vi "AppInit.vi"(10 "path":path, 11 "Changelog":string caption="App Ver") -> (0 "error out":errorcluster)   [LabVIEW 2016]
doc: "Init Host application"
uses:
  tools/Windows/Windows.ExitAction.ctl
  tools/EventLog/EventLog.Buffer.Action.ctl
  tools/Translator/Translator.Message.ctl
  Global/ApplicationGlobal.vi
  Station/Station.Global.vi
  tools/EventLog/EventLog.New(single).vi
  tools/Config/Config.Global.vi
panel:
  out "idx":i32
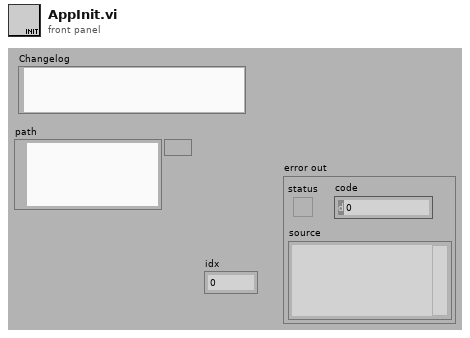
[diagram p1: front panel]
types:
  T1 = enum32{"Invalid", "Standard", "Closed", "Hidden", "Minimized", "Maximized"}
  T2 = typedef "Windows.ExitAction.ctl" = enum16{"Log off from PC", "Shut Down PC", "Reboot PC", "Close Program"}
  T3 = typedef "EventLog.Buffer.Action.ctl" = enum16{"init", "re-init", "clear", "set translator", "add", "get", "get unsaved"}
  T4 = typedef "Translator.Message.ctl" = enum16{"-", "Event confirmed", "Log out", "Log in", "Shutdown", "Cancel", "Start", "Begin time", "End time", "Duration", "Service Mode", "Ignore Results", "Serial Format", "On", "Off", "OK", "NOK", "NOK %s", "Home", "Work", "Close", "Open", "In progress...", "Missing", "Empty", "Hardware failure", "Initial", "Default", "Total", "Out of range", "Free disk space is below 1GB - contact technician", "Error %d >> %s", "Error %d >> %s >> %s", "Msg %d >> %s", "Laser msg %d %s", "Laser cmd error %s %d", "Laser cmd failed %s", "Laser cmd warning %s", "Laser disconnected", "Laser status %s", "Laser already started", "Laser job unkonwn %s", "Laser job missing %s", "Laser job select failure %s", "Unable to start laser printing (%s)", "Unable to stop laser printing (%s)", "Laser marking aborted", "Laser marking timeout", "Unable to reset Laser Interlock (%s)", "Unable to trigger Laser. Laser not ready (%s)", "Laser job '%s' coordinates not configured", "Starting %s", "Quitting %s", "Configured", "Initializing", "Quitting", "Loading", "Loaded %d results", "Loaded %d events", "Running", "Stopped", "Summary", "Laser", "Do you want to continue?", "Do you want to delete the configuration?", "The configuration is being used by an order. Unable to delete!", "Press confirm button", "Station is not based. Do you want to exit?", "Station requires changeover. Do you want to run the test?", "Test options are not set as default. Do you want to continue?", "Formatting of WabcoNo is disabled. Do you want to continue?", "Product not detected. Do you want to continue?", "Product scan failed. Do you want to continue?", "Calibration", "Log out?", "System", "All", "IDLE", "Translating...%s", "Not found", "Alarm %s", "Run", "Skip", "Abort", "Repeat", "Please wait...", "Database disconnected", "Database disconnected - changeover disabled!", "Login to database successful", "Login to database failed: %d; %s", "Unable to check the product status of reference %d - database disconnected", "Unable to set the product status of reference %d - database disconnected", "Variant file backup %s", "Read variant (%s)", "Result", "Station armed!", "Station requires changeover!", "Select reference number...", "EMERGENCY BUTTON - press Control button", "EMERGENCY DOOR - press Control button", "Resetting Emergency...", "Unable to reset safety circuit - Emergency Button pressed", "Unable to reset safety circuit - Emergency Side Door open", "Station not based", "Station based", "Station not empty", "Station basing...", "No order", "Press Start to begin new order", "Scanning new order", "Order NOK. Correct or scan again", "Order OK. Press Accept", "Order ready", "Revolver incorrect", "Fork incorrect", "Revolver missing", "Revolver empty", "Container missing", "Offline results", "Offline statistics", "Updating statistics %.1f %%", "DMC Configurator", "Door open", "Close the front door", "Press start button", "Done. Open the front door", "Running...", "Running...%.1f %%", "Pause %s", "Pause %s. NOK container missing", "Pause %s. OK container missing", "Pause %s. Revolver empty", "Pause %s. Revolver missing", "Pause %s. Revolver incorrect", "Pause %s. Fork missing", "Pause %s. Fork incorrect", "Pause %s. Too many failures", "Pause %s. Unloading failure", "Pause %s. One slot is not working", "Pause %s. Part order is done. Empty OK container", "Pause %s. Unable to move product to slot", "Pause %s. Unable to move back product pusher", "Pause %s. Unable to lift product", "Pause %s. Unable to move back product lifter", "Pause %s. Unable to move product arm to Work", "Pause %s. Unable to move product arm to NOK", "Pause %s. Unable to move product arm to OK", "Pause %s. Unable to unsuck the NOK product", "Pause %s. Unable to drop the NOK product", "Pause %s. Product OK missing", "Pause %s. Unable to unsuck the OK product", "Pause %s. Unable to drop the OK product", "Stopping...", "File '%s' is missing", "File '%s' is broken", "File '%s' is running", "Log file started (%s)", "Log file ended (%s)", "Log file stopped (%s)", "Log file ignored (%s)", "Log file exported (%s)", "Log file export failed (%s)", "Wrong serial number in log file", "Wrong reference number in log file", "Test steps are missing", "%s = %.3f", "Process param '%s' not found in DB", "Process param '%s' wrong order", "Process param '%s' value %.3f out of limits (%.3f; %.3f)", "Step%d param '%s' not found in DB", "Step%d param '%s' wrong order", "Step%d param '%s' value %.3f out of limits (%.3f; %.3f)", "Step%d EV '%s' not found in DB", "Step%d EV '%s' wrong order", "\"%s\" not found in DB", "\"%s\" wrong order", "\"%s\" value %.3f out of limits (%.3f; %.3f)", "\"%s\" not found in software", "Process init (%s)", "Process started", "Process restarted", "Process run", "Process done", "Process done - remove OK container", "Process aborted", "Process aborted at work", "Process aborted at home", "Process error", "Process error at home", "Process error at work", "Process close", "Process pause", "Process continue", "Process door open", "Process door close", "Process pause at slot %s due to %s", "Select plate from the order to process", "Do you want to start the process?", "Do you want to continue the process?", "There is unfinished order. Do you want to put the new order?", "Product %s %d OK", "Product %s %d NOK", "Unable to unload the slot %s. Product missing in the slot", "Unable to unload the slot %s. Product already in the arm", "Unable to accept the product as OK. Product missing in slot %s", "Unable to accept the product as OK. Product could not drop into the container at slot %s", "Unable to accept the product as NOK. Product could not drop into the container at slot %s", "Scan failed. Error %s", "Scan failed. Scanner disconnected", "Scan failed. Wrong Wabco number %d, limit (%d,%d)", "Scan failed. Wrong serial number %d, limit (%d,%d)", "Scan failed. Wrong date %d, limit (%d,%d)", "Scan failed. Wrong product wabco number %d (expected %d)", "Scan failed. Wrong product serial number %d (expected > 0)", "Scan OK %s", "Scan failed. Unable to determine table position (%s)", "Scan failed. Timeout", "Tune failed. Scanner disconnected", "Tune failed. Timeout", "%s = %d", "%s = %d->%d", "Unable to set %s = %.2f - Air Pressure Inside off", "Unable to set digital output '%s' = %d", "Unable to activate air pressure inside - timeout", "Unable to activate air pressure inside - aborted", "Unable to switch on Air Main Valve - Air Pressure Inlet off", "Unable to switch on Air Main Valve - Door open", "Unable to switch off Air Main Valve - timeout", "Unable to switch off Air Main Valve - aborted", "Unable to rotate Table - timeout", "Unable to rotate Table - aborted", "Unable to rotate Table - Product Move not in Home position", "Unable to rotate Table - Air Pressure Inside off", "Unable to rotate Table - Product Lift A not in Home position", "Unable to rotate Table - Product Lift B not in Home position", "Unable to rotate Table - unlock before movement timeout", "Unable to rotate Table - lock after movement timeout", "Unable to move Table Lock to %s position - timeout", "Unable to move Table Lock to %s position - aborted", "Unable to move Table Lock to %s position - Air Pressure Inside off", "Unable to move Table Lock to %s position - Table not in position", "Unable to move Product Lift A to %s position - timeout", "Unable to move Product Lift B to %s position - timeout", "Unable to move Product Lift A to %s position - aborted", "Unable to move Product Lift B to %s position - aborted", "Unable to move Product Lift A to %s position - Air Pressure Inside off", "Unable to move Product Lift B to %s position - Air Pressure Inside off", "Unable to move Product Lift A to %s position - Table not locked", "Unable to move Product Lift B to %s position - Table not locked", "Unable to move Product Lift A to %s position - Product Arm not in Work position", "Unable to move Product Lift B to %s position - Product Arm not in Work position", "Unable to set Product Suction Gripper %s to %s - timeout", "Unable to set Product Suction Gripper %s to %s - aborted", "Unable to set Product Suction Gripper %s to %s - Air Pressure Inside off", "Unable to set Product Suction Gripper %s to %s - Table slot unkown", "Unable to move Product Arm to %s position - timeout", "Unable to move Product Arm to %s position - aborted", "Unable to move Product Arm to %s position - Air Pressure Inside off", "Unable to move Product Arm to %s position - Product Lift A not in Home position", "Unable to move Product Arm to %s position - Product Lift B not in Home position", "Unable to move Product to %s position - timeout", "Unable to move Product to %s position - aborted", "Unable to move Product to %s position - Air Pressure Inside off", "Unable to move Product to %s position - Table not in position"}
  T5 = enum32{"invalid app kind", "Development System", "Run Time System", "Student Edition", "Embedded LabVIEW", "Evaluation", "Custom"}
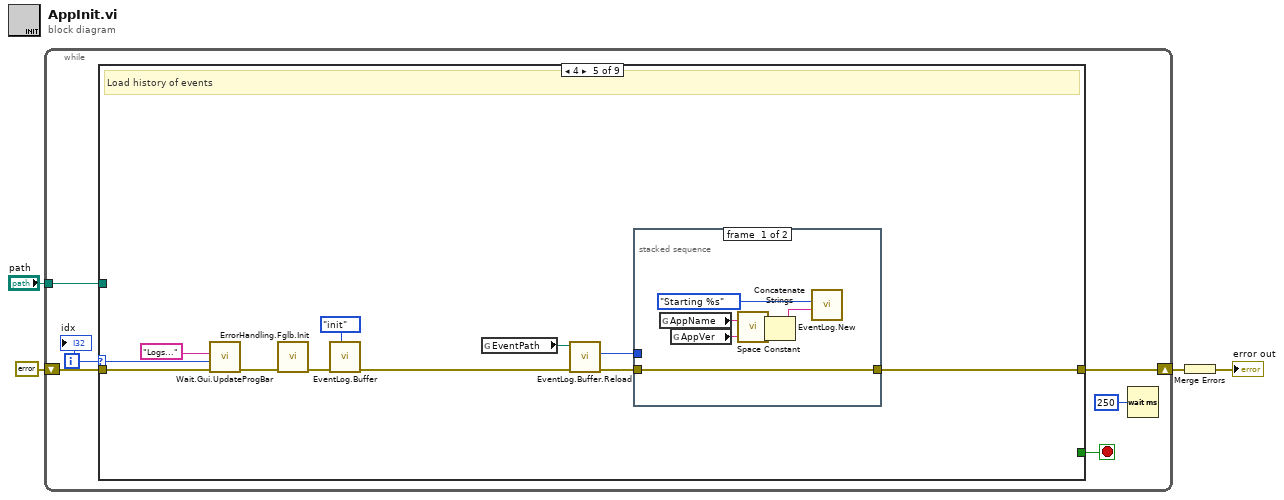
[diagram p0: block diagram]
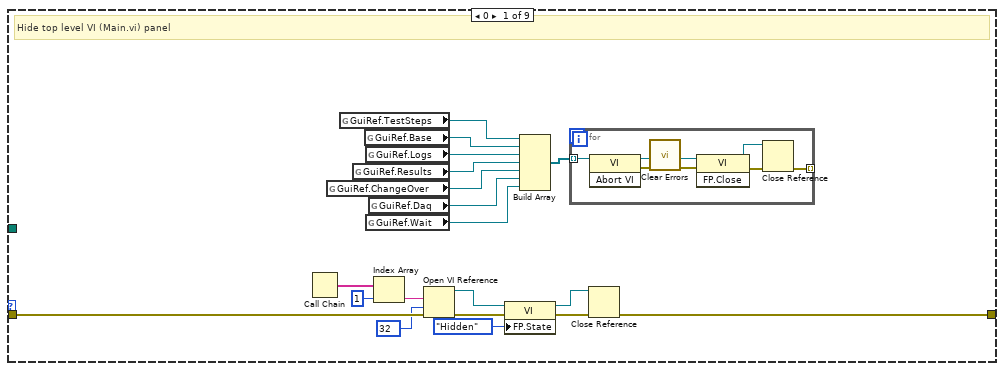
[diagram p2: hidden frame]
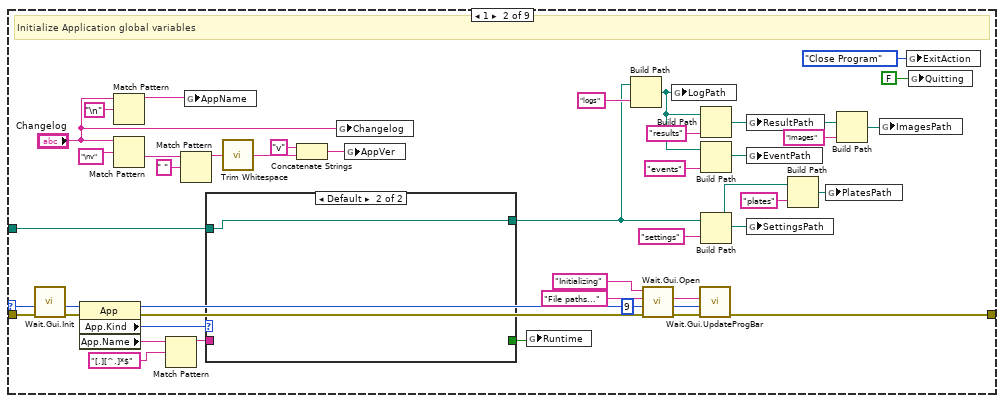
[diagram p3: hidden frame]
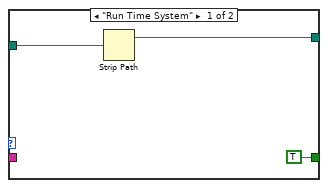
[diagram p4: hidden frame]
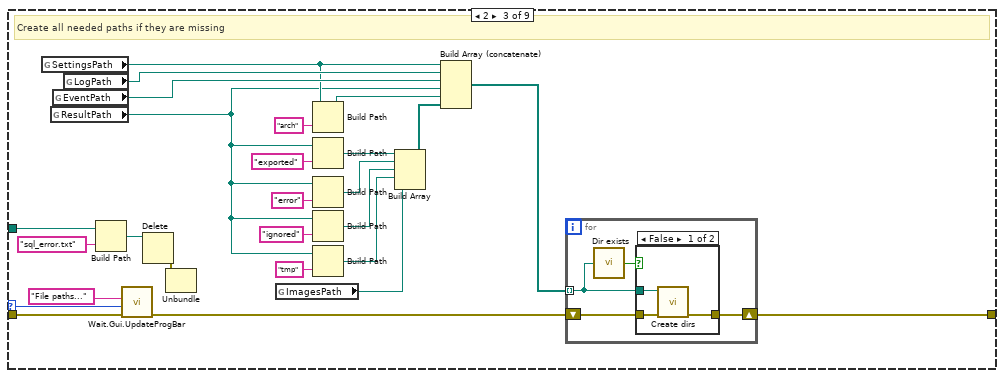
[diagram p5: hidden frame]
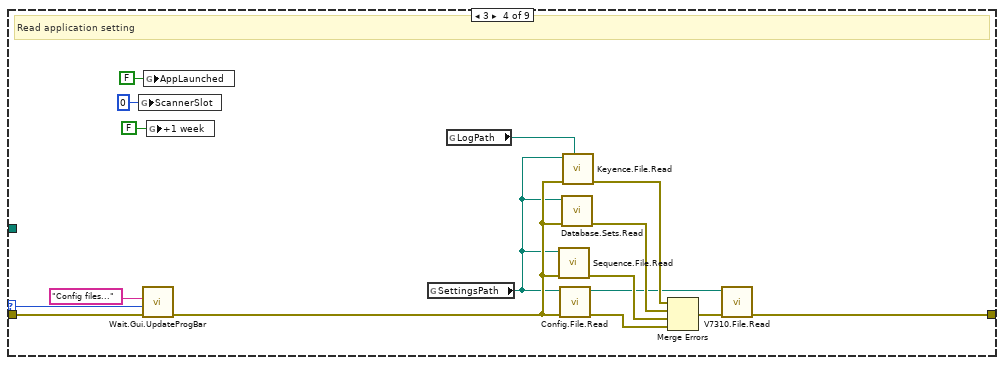
[diagram p7: hidden frame]
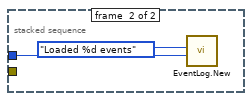
[diagram p8: hidden frame]
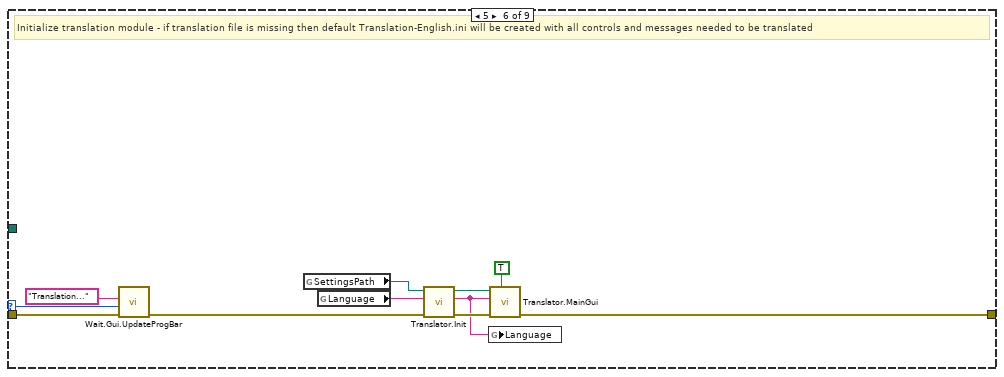
[diagram p9: hidden frame]
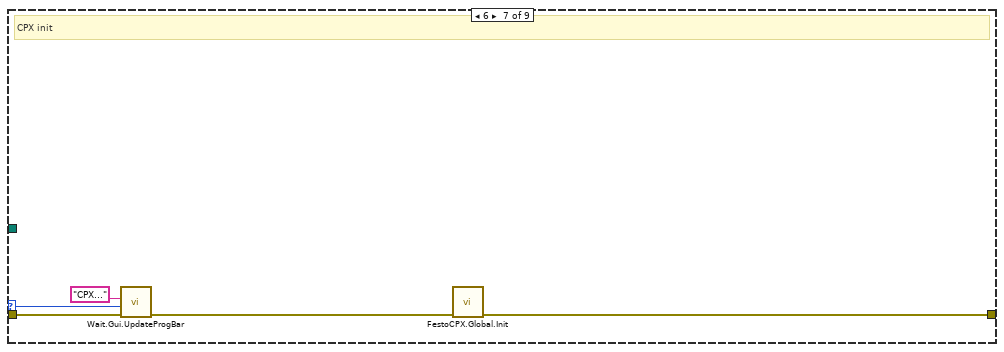
[diagram p10: hidden frame]
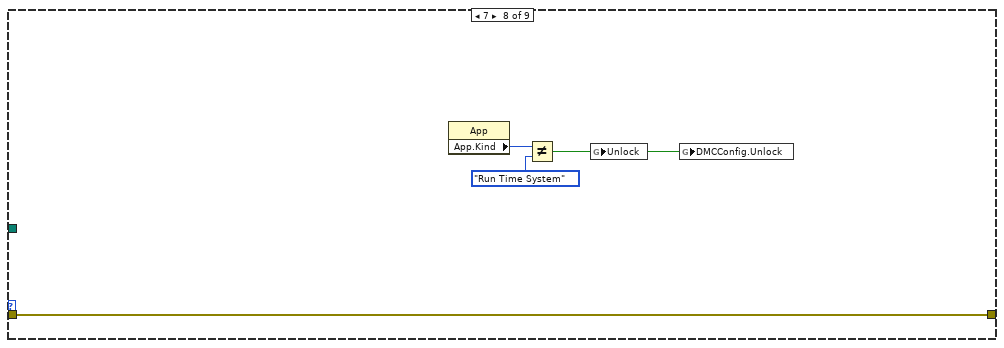
[diagram p11: hidden frame]
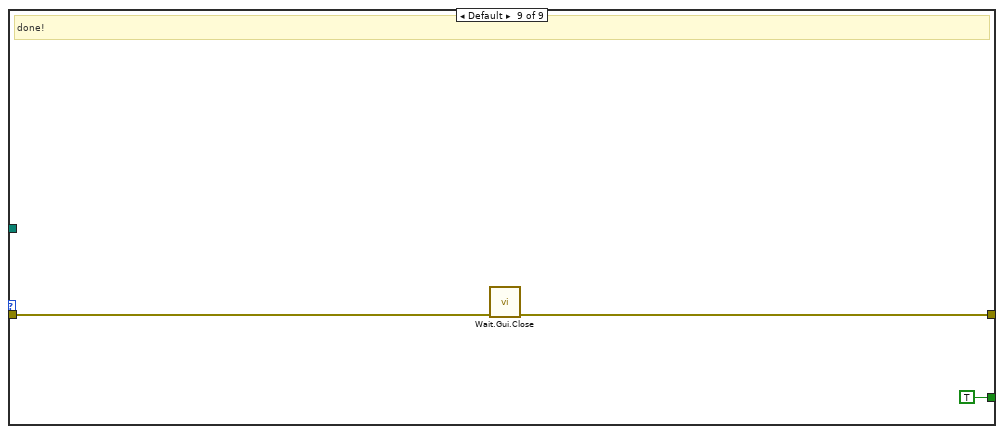
[diagram p12: hidden frame]
diagram:
  n1 = while {
    shift-right: [w8] -> w3
    shift-left: errorcluster {"status"=FALSE, "code"=0, "source"=""} ("error out") -> [w10]
    tunnel: "path" -> [w7]
    i -> [w6]
    stop <- w9 stop-if-true
    n2 = case shown="4" w6 {
      selector: w6 -> [_ w45 w94 w128 w133 w151 w161 _ _]
      tunnel: w10 -> [w28 w42 w93 w127 w132 w152 w160 w167 w169]
      tunnel: [_ _ _ _ _ _ _ _ TRUE] -> w9
      tunnel: [w14 w46 w104 w118 w138 w150 w163 w167 w168] -> w8
      tunnel: w7 -> [_ w55 w89 _ _ _ _ _ _]
      frame 0 {
        # "Hide top level VI (Main.vi) panel"
        n3 = Call Chain() -> (call chain=w23:string[])
        n4 = global read "ApplicationGlobal.vi" "GuiRef.ChangeOver"() -> (w16:refnum<vi>)
        n5 = global read "ApplicationGlobal.vi" "GuiRef.TestSteps"() -> (w12:refnum<vi>)
        n6 = global read "ApplicationGlobal.vi" "GuiRef.Results"() -> (w17:refnum<vi>)
        n7 = global read "ApplicationGlobal.vi" "GuiRef.Base"() -> (w19:refnum<vi>)
        n8 = global read "ApplicationGlobal.vi" "GuiRef.Logs"() -> (w18:refnum<vi>)
        n9 = global read "ApplicationGlobal.vi" "GuiRef.Wait"() -> (w11:refnum<vi>)
        n10 = global read "ApplicationGlobal.vi" "GuiRef.Daq"() -> (w13:refnum<vi>)
        n11 = Index Array(array=w23, index=1) -> (element=w21:string)
        n12 = Open VI Reference(vi path=w21, options=32, error in (no error)=w28) -> (vi reference=w26:refnum<vi>, error out=w27:errorcluster)  [unwired: 3 in]
        n13 = property class="VI"(reference=w26, error in=w27, "FP.State"=T1."Hidden" ("Front Panel Window:State")) -> (reference out=w24:refnum<vi>, error out=w25:errorcluster)
        n14 = Build Array(w12, w19, w18, w17, w16, w13, w11) -> (w15:refnum<vi>[])
        n15 = for {
          tunnel: w15 -> [w33] mode=indexing
          tunnel: [w34] -> _ mode=indexing
          n16 = invoke class="VI" method="Abort VI"(reference=w33) -> (reference out=w32:refnum<vi>, error out=w31:errorcluster)  [unwired: 2 in, 1 out]
          n17 = call <vilib>:"Clear Errors.vi"("error in (no error)"=w31) -> ("error out"=w30:errorcluster)  [unwired: 5 in, 1 out]
          n18 = invoke class="VI" method="FP.Close"(reference=w32, error in=w30) -> (reference out=w36:refnum<vi>, error out=w35:errorcluster)  [unwired: 1 in, 1 out]
          n19 = Close Reference(reference=w36, error in (no error)=w35) -> (error out=w34:errorcluster)
        }
        n20 = Close Reference(reference=w24, error in (no error)=w25) -> (error out=w14:errorcluster)
      }
      frame 1 {
        w49 = "File paths..."
        # "Initialize Application global variables"
        n21 = call "Wait.Gui.Init.vi"("error in (no error)"=w42) -> ("error out"=w41:errorcluster)  [unwired: 10 in]
        n22 = property class="App"(error in=w41) -> (error out=w47:errorcluster, "App.Kind"=w68:T5, "App.Name"=w62:string)  [unwired: 1 in, 1 out]
        n23 = Match Pattern(string="Changelog", regular expression="\n") -> (before substring=w53:string)  [unwired: 1 in, 3 out]
        n24 = Match Pattern(string="Changelog", regular expression="\nv") -> (after substring=w74:string)  [unwired: 1 in, 3 out]
        n25 = Match Pattern(string=w62, regular expression="[.][^.]*$") -> (before substring=w61:string)  [unwired: 4 out]
        n26 = Match Pattern(string=w74, regular expression=" ") -> (before substring=w71:string)  [unwired: 1 in, 3 out]
        n27 = global write "ApplicationGlobal.vi" "AppName"(w53) -> ()
        n28 = case shown="Default" w68 {
          tunnel: [w79 w80] -> w51
          tunnel: w61 -> [_ _]
          tunnel: w55 -> [w78 w80]
          tunnel: [TRUE ("Quitting") _] -> w40
          frame "Run Time System" {
            n29 = Strip Path(path=w78) -> (stripped path=w79:path)  [unwired: 1 out]
          }
          frame Default {
          }
        }
        n30 = call <vilib>:"Trim Whitespace.vi"("string"=w71) -> ("trimmed string"=w69:string)  [unwired: 1 in]
        n31 = Concatenate Strings("v" ("string"), w69) -> (w52:string)
        n32 = global write "ApplicationGlobal.vi" "Changelog"("Changelog") -> ()
        n33 = global write "ApplicationGlobal.vi" "AppVer"(w52) -> ()
        n34 = global write "ApplicationGlobal.vi" "Runtime"(w40) -> ()
        n35 = Build Path(base path=w51, name or relative path="logs") -> (appended path=w58:path)
        n36 = call "Wait.Gui.Open.vi"("error in (no error)"=w47, "ProgBarSize (0)"=9 ("ProgBarSize"), "Status (\"\")"=w49, "Msg"="Initializing" ("format string")) -> ("error out"=w50:errorcluster)  [unwired: 7 in]
        n37 = global write "ApplicationGlobal.vi" "LogPath"(w58) -> ()
        n38 = call "Wait.Gui.UpdateProgBar.vi"("error in (no error)"=w50, "ProgBar (0)"=w45, "status (\"\")"=w49) -> ("error out"=w46:errorcluster)  [unwired: 8 in]
        n39 = Build Path(base path=w58, name or relative path="results") -> (appended path=w38:path)
        n40 = Build Path(base path=w58, name or relative path="events") -> (appended path=w65:path)
        n41 = Build Path(base path=w51, name or relative path="settings") -> (appended path=w44:path)
        n42 = global write "ApplicationGlobal.vi" "ResultPath"(w38) -> ()
        n43 = global write "ApplicationGlobal.vi" "EventPath"(w65) -> ()
        n44 = global write "ApplicationGlobal.vi" "SettingsPath"(w44) -> ()
        n45 = Build Path(base path=w44, name or relative path="plates") -> (appended path=w57:path)
        n46 = global write "ApplicationGlobal.vi" "PlatesPath"(w57) -> ()
        n47 = Build Path(base path=w38, name or relative path="images") -> (appended path=w37:path)
        n48 = global write "ApplicationGlobal.vi" "ImagesPath"(w37) -> ()
        n49 = global write "ApplicationGlobal.vi" "ExitAction"(Windows.ExitAction."Close Program" ("ExitAction")) -> ()
        n50 = global write "ApplicationGlobal.vi" "Quitting"(FALSE ("Quitting")) -> ()
      }
      frame 2 {
        # "Create all needed paths if they are missing"
        n51 = global read "ApplicationGlobal.vi" "SettingsPath"() -> (w86:path)
        n52 = global read "ApplicationGlobal.vi" "ResultPath"() -> (w82:path)
        n53 = global read "ApplicationGlobal.vi" "EventPath"() -> (w105:path)
        n54 = global read "ApplicationGlobal.vi" "LogPath"() -> (w106:path)
        n55 = Build Path(base path=w89, name or relative path="sql_error.txt") -> (appended path=w90:path)
        n56 = call "Wait.Gui.UpdateProgBar.vi"("error in (no error)"=w93, "ProgBar (0)"=w94, "status (\"\")"="File paths...") -> ("error out"=w92:errorcluster)  [unwired: 8 in]
        n57 = Delete(path (use dialog)=w90) -> (error out=w88:errorcluster)  [unwired: 4 in, 2 out]
        n58 = Unbundle(w88) -> ()  [unwired: 3 out]
        n59 = global read "ApplicationGlobal.vi" "ImagesPath"() -> (w84:path)
        n60 = Build Path(base path=w86, name or relative path="arch") -> (appended path=w85:path)
        n61 = Build Path(base path=w82, name or relative path="exported") -> (appended path=w99:path)
        n62 = Build Path(base path=w82, name or relative path="error") -> (appended path=w97:path)
        n63 = Build Path(base path=w82, name or relative path="ignored") -> (appended path=w98:path)
        n64 = Build Path(base path=w82, name or relative path="tmp") -> (appended path=w81:path)
        n65 = Build Array(w99, w97, w98, w81, w84) -> (w96:path[])
        n66 = Build Array (concatenate)(w86, w106, w105, w82, w85, w96) -> (w103:path[])
        n67 = for {
          tunnel: w103 -> [w108] mode=indexing
          shift-right: [w109] -> w104
          shift-left: w92 -> [w110]
          n68 = call "Dir exists.vi"("dir path"=w108) -> ("exists?"=w107:bool)  [unwired: 4 in]
          n69 = case shown="False" w107 {
            tunnel: w108 -> [w113 _]
            tunnel: w110 -> [w112 w114]
            tunnel: [w111 w114] -> w109
            frame False {
              n70 = call "Create dirs.vi"("error in (no error)"=w112, "deepest dir"=w113) -> ("error"=w111:errorcluster)  [unwired: 9 in]
            }
            frame True {
            }
          }
        }
      }
      frame 3 {
        # "Read application setting"
        n71 = global write "Station.Global.vi" "ScannerSlot"(0 ("ScannerSlot")) -> ()
        n72 = call "Wait.Gui.UpdateProgBar.vi"("error in (no error)"=w127, "ProgBar (0)"=w128, "status (\"\")"="Config files...") -> ("error out"=w120:errorcluster)  [unwired: 8 in]
        n73 = global write "ApplicationGlobal.vi" "AppLaunched"(FALSE ("AppLaunched")) -> ()
        n74 = global write "Station.Global.vi" "+1 week"(FALSE ("+1 week")) -> ()
        n75 = global read "ApplicationGlobal.vi" "SettingsPath"() -> (w116:path)
        n76 = global read "ApplicationGlobal.vi" "LogPath"() -> (w125:path)
        n77 = call "Sequence.File.Read.vi"("error in"=w120, "path"=w116) -> ("error out"=w123:errorcluster)  [unwired: 8 in, 1 out]
        n78 = call "Config.File.Read.vi"("error in"=w120, "path"=w116) -> ("error out"=w117:errorcluster)  [unwired: 9 in]
        n79 = call "Database.Sets.Read.vi"("error in"=w120, "SettingsPath"=w116) -> ("error out"=w119:errorcluster)  [unwired: 9 in]
        n80 = call "Keyence.File.Read.vi"("log path"=w125, "error in"=w120, "segtings path"=w116) -> ("error out"=w124:errorcluster)  [unwired: 8 in]
        n81 = Merge Errors(w124, w119, w123, w117) -> (w115:errorcluster)
        n82 = call "V7310.File.Read.vi"("error in"=w115, "SettingsPath"=w116) -> ("error out"=w118:errorcluster)  [unwired: 9 in]
      }
      frame 4 {
        # "Load history of events"
        n83 = call "Wait.Gui.UpdateProgBar.vi"("error in (no error)"=w132, "ProgBar (0)"=w133, "status (\"\")"="Logs...") -> ("error out"=w130:errorcluster)  [unwired: 8 in]
        n84 = call "ErrorHandling.Fglb.Init.vi"("error in (no error)"=w130) -> ("error out"=w135:errorcluster)  [unwired: 10 in]
        n85 = call "EventLog.Buffer.vi"("action (get)"=EventLog.Buffer.Action."init" ("action (read)"), "error in"=w135) -> ("error out"=w136:errorcluster)  [unwired: 6 in, 3 out]
        n86 = global read "ApplicationGlobal.vi" "EventPath"() -> (w140:path)
        n87 = call "EventLog.Buffer.Reload.vi"("error in"=w136, "Path"=w140) -> ("error out"=w139:errorcluster, "#loaded entries"=w131:i32)  [unwired: 8 in]
        n88 = stacked-sequence {
          tunnel: [w145 _] -> w138
          tunnel: w139 -> [w145 _]
          tunnel: w131 -> [_ w147]
          frame #0 {
            n89 = global read "ApplicationGlobal.vi" "AppName"() -> (w144:string)
            n90 = global read "ApplicationGlobal.vi" "AppVer"() -> (w143:string)
            n91 = call <vilib>:"Space Constant.vi"() -> ("String"=w142:string)
            n92 = Concatenate Strings(w144, w142, w143) -> (w141:string)
            n93 = call-poly "EventLog.New.vi"("Arg"=w141, "Message (-)"=Translator.Message."Starting %s") -> ()  [unwired: 8 in, 2 out]
          }
          frame #1 {
            n94 = call-poly "EventLog.New.vi"("Arg"=w147, "Message (-)"=Translator.Message."Loaded %d events") -> ()  [unwired: 8 in, 2 out]
          }
        }
      }
      frame 5 {
        # "Initialize translation module - if translation file is missing then default Translation-English.ini will be created with all controls and messages needed to be translated"
        n95 = call "Wait.Gui.UpdateProgBar.vi"("error in (no error)"=w152, "ProgBar (0)"=w151, "status (\"\")"="Translation...") -> ("error out"=w149:errorcluster)  [unwired: 8 in]
        n96 = global read "ApplicationGlobal.vi" "SettingsPath"() -> (w156:path)
        n97 = global read "Config.Global.vi" "Language"() -> (w157:string)
        n98 = call "Translator.Init.vi"("error in"=w149, "Language in"=w157, "Translation folder"=w156) -> ("error out"=w158:errorcluster, "Language out"=w155:string)  [unwired: 7 in]
        n99 = global write "Config.Global.vi" "Language"(w155) -> ()
        n100 = call "Translator.MainGui.vi"("~init (F)"=TRUE ("init (F)"), "~error in"=w158, "~Language in use"=w155, "~Translation folder"=w156) -> ("~error out"=w150:errorcluster)  [unwired: 4 in, 3 out]
      }
      frame 6 {
        # "CPX init"
        n101 = call "Wait.Gui.UpdateProgBar.vi"("error in (no error)"=w160, "ProgBar (0)"=w161, "status (\"\")"="CPX...") -> ("error out"=w159:errorcluster)  [unwired: 8 in]
        n102 = call "FestoCPX.Global.Init.vi"("error in (no error)"=w159) -> ("error out"=w163:errorcluster)  [unwired: 10 in]
      }
      frame 7 {
        n103 = property class="App"() -> ("App.Kind"=w166:T5)  [unwired: 2 in, 2 out]
        n104 = Not Equal?(x=w166, y=T5."Run Time System") -> (x != y?=w164:bool)
        n105 = global write "ApplicationGlobal.vi" "Unlock"(w164) -> ()
        n106 = global write "ApplicationGlobal.vi" "DMCConfig.Unlock"(w164) -> ()
      }
      frame Default {
        # "done!"
        n107 = call "Wait.Gui.Close.vi"("error in (no error)"=w169) -> ("error out"=w168:errorcluster)  [unwired: 10 in]
      }
    }
    n108 = Wait (ms)(milliseconds to wait=u32 250) -> ()  [unwired: 1 out]
    "idx" <- w6
  }
  n109 = Merge Errors(w3) -> (→"error out":errorcluster)
